vi "Teleop.vi"(10 "Match Info":T1={"Autonomous Elapsed Seconds"=0.0, "TeleOp Elapsed Seconds"=0.0, "Disabled Elapsed Seconds"=0.0, "Visited Autonomous"=FALSE, "Visited TeleOp"=FALSE, "Visited Disabled"=FALSE, "Autonomous Settings"={"Autonomous Style"=enum."Independent", "VI Refnum"=refnum}}, 11 "Call Context":T2) -> ()   [LabVIEW 2019]
doc: "This VI is called for each TeleOp packet received from the DS where the robot is not disabled. It is often used to read from the joysticks and update I/O or to update setpoints for timed control loops. It should complete and return within 20 milliseconds or it may miss DS packets."
uses:
  <vilib>/Rock Robotics/WPI/DriverStation/WPI_DriverStationDerivedRobotMode.ctl
  <vilib>/Rock Robotics/WPI/DriverStation/WPI_DriverStationMatch Info.ctl
  <vilib>/Rock Robotics/WPI/ThirdParty/Phoenix-LabVIEW/Motor Controller/Controls/CTRE_Phoenix_MotorControl_ControlMode.ctl
  <vilib>/Rock Robotics/WPI/Solenoid/WPI_SolenoidValue.ctl
  <vilib>/Rock Robotics/WPI/Utilities/WPI_GetSetVariantRefNum.vi
  <vilib>/Rock Robotics/Network Tables/NT Read Boolean.vi
  <vilib>/Rock Robotics/Network Tables/NT Read Number.vi
  <vilib>/Rock Robotics/WPI/Solenoid/WPI_SolenoidSetEnum.vi
  <vilib>/Rock Robotics/WPI/RobotDrive/WPI_RobotDriveMecanumDrive_Cartesian.vi
  <vilib>/Rock Robotics/Network Tables/NT Write Numeric Array.vi
panel:
  out "Sample Slider 0":dbl(slide) scale=0.0..5.0
  out "Sample Boolean 1":bool
  out "Sample Boolean 0":bool
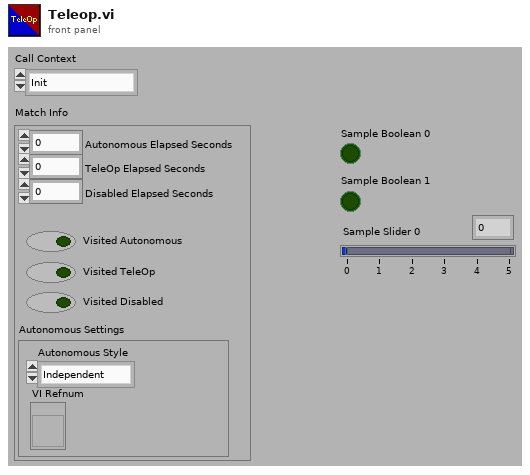
[diagram p1: front panel]
types:
  T1 = typedef "WPI_DriverStationMatch Info.ctl" = cluster{"Autonomous Elapsed Seconds":dbl, "TeleOp Elapsed Seconds":dbl, "Disabled Elapsed Seconds":dbl, "Visited Autonomous":bool, "Visited TeleOp":bool, "Visited Disabled":bool, "Autonomous Settings":cluster{"Autonomous Style":enum16{"Iterative", "Independent"}, "VI Refnum":refnum<vi>}}
  T2 = typedef "WPI_DriverStationDerivedRobotMode.ctl" = enum16{"Init", "Execute", "Stop"}
  T3 = typedef "CTRE_Phoenix_MotorControl_ControlMode.ctl" = u16
  T4 = typedef "WPI_JoystickDevRef.ctl" = cluster{"Device":T5}
  T5 = typedef "WPI_JoystickDeviceEnum.ctl" = enum16{"USB 0", "USB 1", "USB 2", "USB 3", "USB 4", "USB 5"}
  T6 = typedef "WPI_DigitalInputDevRef.ctl" = cluster{"DevStatus":errorcluster, "DIO Channel":T7}
  T7 = typedef "FPGA_DIOChannel.ctl" = enum8{"DIO 0", "DIO 1", "DIO 2", "DIO 3", "DIO 4", "DIO 5", "DIO 6", "DIO 7", "DIO 8", "DIO 9", "DIO MXP 0", "DIO MXP 1", "DIO MXP 2", "DIO MXP 3", "DIO MXP 4", "DIO MXP 5", "DIO MXP 6", "DIO MXP 7", "DIO MXP 8", "DIO MXP 9", "DIO MXP 10", "DIO MXP 11", "DIO MXP 12", "DIO MXP 13", "DIO MXP 14", "DIO MXP 15", "SPI Port CS1", "SPI Port CS2", "SPI Port CS3", "SPI Port MISO", "SPI Port MOSI", "Invalid"}
  T8 = typedef "WPI_MotorControlDeviceRef.ctl" = cluster{"DeviceStatus":errorcluster, "Type":T9, "PWM":cluster{"PWM Channel":T10, "DeadBand":T11}, "CAN":cluster{"Device Number":u8, "SetOutput VI Ref":variant, "GetOutput VI Ref":variant, "Enable VI Ref":variant, "Disable VI Ref":variant, "Data":variant}, "Invert":bool, "DIO PWM":cluster{"PWM \"Enable\" Channel":T10, "DIOChannel":T7, "PWM Rate":dbl}}
  T9 = typedef "WPI_MotorControlType.ctl" = enum16{"PWM", "CAN", "DIO PWM"}
  T10 = typedef "FPGA_DIOPWMChannel.ctl" = enum8{"PWM 0", "PWM 1", "PWM 2", "PWM 3", "PWM 4", "PWM 5", "PWM 6", "PWM 7", "PWM 8", "PWM 9", "PWM MXP 0", "PWM MXP 1", "PWM MXP 2", "PWM MXP 3", "PWM MXP 4", "PWM MXP 5", "PWM MXP 6", "PWM MXP 7", "PWM MXP 8", "PWM MXP 9", "Invalid"}
  T11 = typedef "WPI_PWMDeadband.ctl" = cluster{"Name":string, "maxPositivePwm":i32, "minPositivePwm":i32, "centerPwm":i32, "maxNegativePwm":i32, "minNegativePwm":i32, "angularRange":u16}
  T12 = typedef "WPI_RobotDriveDevRef.ctl" = cluster{"DevStatus":errorcluster, "Motors[]":T8[], "Square Inputs":bool, "Max Output":dbl}
  T13 = typedef "WPI_SolenoidDevRef.ctl" = cluster{"DevStatus":errorcluster, "Pneumatics Control Module":u8, "Forward Solenoid Channel":T14, "Reverse Solenoid Channel":T14}
  T14 = typedef "WPI_SolenoidChannel.ctl" = enum8{"Solenoid 0", "Solenoid 1", "Solenoid 2", "Solenoid 3", "Solenoid 4", "Solenoid 5", "Solenoid 6", "Solenoid 7", "Invalid"}
  T15 = typedef "WPI_SolenoidValue.ctl" = enum16{"Off", "On", "Forward", "Reverse"}
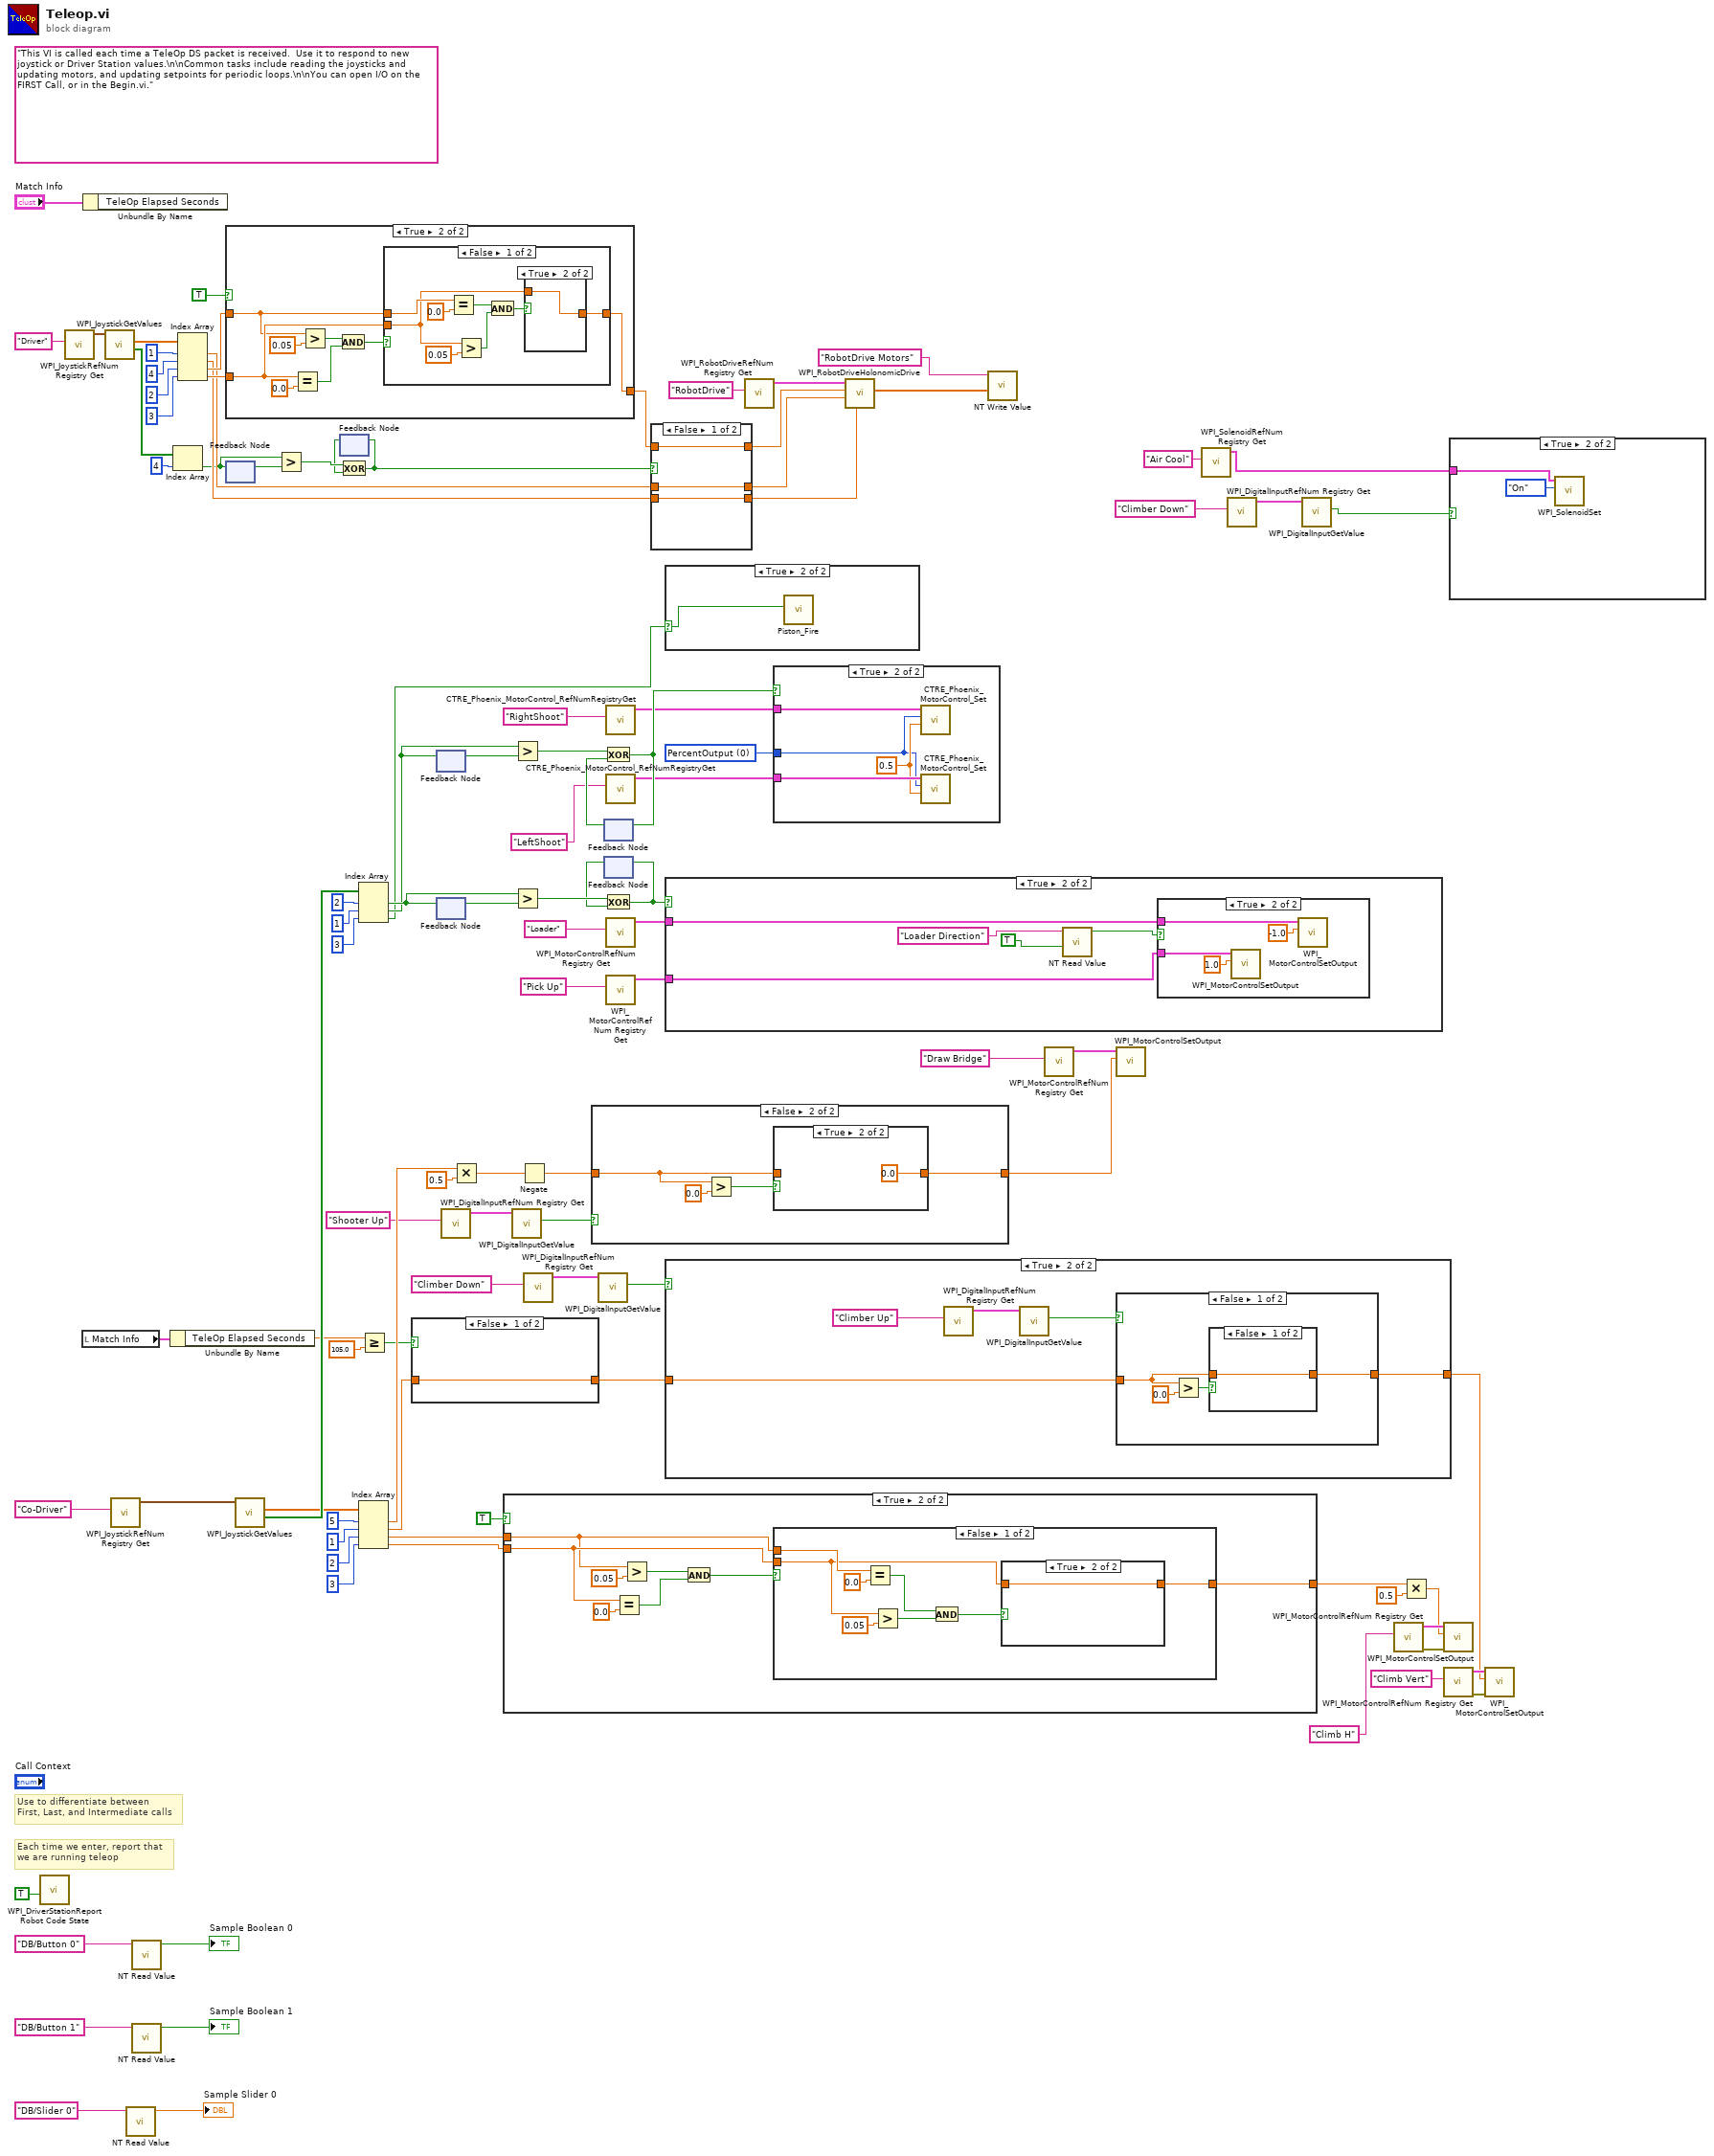
[diagram p0: block diagram]
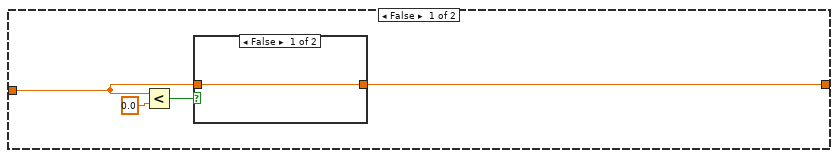
[diagram p3: hidden frame]
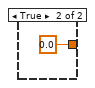
[diagram p4: hidden frame]
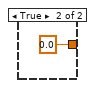
[diagram p5: hidden frame]
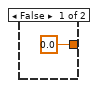
[diagram p10: hidden frame]
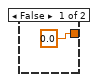
[diagram p11: hidden frame]
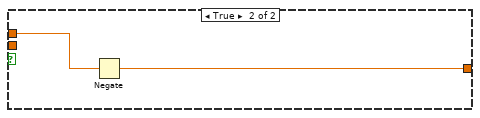
[diagram p12: hidden frame]
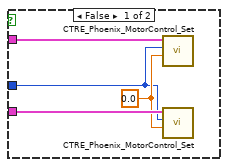
[diagram p14: hidden frame]
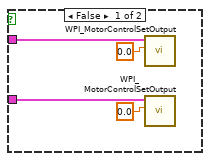
[diagram p15: hidden frame]
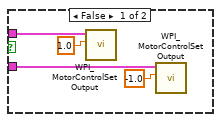
[diagram p16: hidden frame]
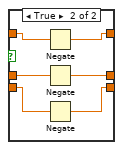
[diagram p17: hidden frame]
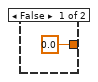
[diagram p18: hidden frame]
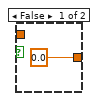
[diagram p19: hidden frame]
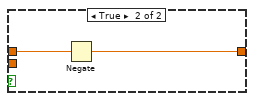
[diagram p20: hidden frame]
diagram:
  w47 = T3 0 items=["PercentOutput"=0, "Position"=1, "Velocity"=2, "Current"=3, "Follower"=5, "MotionProfile"=6, "MotionMagic"=7, "MotionProfileArc"=10, "Disabled"=15] ("Control Mode")
  (unwired) "This VI is called each time a TeleOp DS packet is received.  Use it to respond to new joystick or Driver Station values.\n\nCommon tasks include reading the joysticks and updating motors, and updating setpoints for periodic loops.\n\nYou can open I/O on the FIRST Call, or in the Begin.vi."
  # "Each time we enter, report that\nwe are running teleop"
  # "Use to differentiate between\nFirst, Last, and Intermediate calls"
  n1 = call <vilib>:"WPI_DriverStationReport Robot Code State.vi"("TeleOp"=TRUE ("Autonomous")) -> ()  [unwired: 10 in, 1 out]
  n2 = call <vilib>:"WPI_JoystickRefNum Registry Get.vi"("refnum name"="Driver") -> ("JoystickDevRef"=w99:T4)  [unwired: 1 in, 9 out]
  n3 = local read "Match Info"() -> (w27:T1)
  n4 = Unbundle By Name("Match Info") -> ()  [unwired: 1 out]
  n5 = call <vilib>:"WPI_JoystickGetValues.vi"("JoystickDevRef"=w99) -> ("Buttons"=w75:bool[], "Axes"=w97:dbl[])  [unwired: 6 in, 3 out]
  n6 = call <vilib>:"WPI_JoystickRefNum Registry Get.vi"("refnum name"="Co-Driver") -> ("JoystickDevRef"=w67:T4)  [unwired: 9 in, 1 out]
  n7 = call-poly <vilib>:"NT Read Value.vi"("Name"="DB/Slider 0" ("refnum name")) -> ("Numeric"=→"Sample Slider 0":dbl)  [unwired: 9 in, 1 out]
  n8 = call-poly <vilib>:"NT Read Value.vi"("Name"="DB/Button 0" ("refnum name")) -> ("Boolean"=→"Sample Boolean 0":bool)  [unwired: 9 in, 1 out]
  n9 = call-poly <vilib>:"NT Read Value.vi"("Name"="DB/Button 1" ("refnum name")) -> ("Boolean"=→"Sample Boolean 1":bool)  [unwired: 9 in, 1 out]
  n10 = Unbundle By Name(w27) -> ("TeleOp Elapsed Seconds"=w26:dbl)
  n11 = Index Array(array=w75, index=4) -> (element=w73:bool)
  n12 = Index Array(array=w97, index #1=1 ("index"), index #2=4 ("index"), index #3=2 ("index"), index #4=3 ("index")) -> (element #1=w80:dbl, element #2=w79:dbl, element #3=w83:dbl, element #4=w82:dbl)
  n13 = case shown="True" TRUE {
    tunnel: w83 -> [_ w106]
    tunnel: w82 -> [_ w107]
    tunnel: [0.0 w105] -> w81
    frame False {
    }
    frame True {
      n14 = Equal?(x=w107, y=0.0) -> (x = y?=w109:bool)
      n15 = Greater?(x=w106, y=0.05) -> (0:w110:bool)
      n16 = And(x=w110, y=w109) -> (x .and. y?=w108:bool)
      n17 = case shown="False" w108 {
        tunnel: w107 -> [w114 _]
        tunnel: w106 -> [w120 w124]
        tunnel: [w113 w123] -> w105
        frame False {
          n18 = Equal?(x=w120, y=0.0) -> (x = y?=w117:bool)
          n19 = Greater?(x=w114, y=0.05) -> (0:w116:bool)
          n20 = And(x=w117, y=w116) -> (x .and. y?=w115:bool)
          n21 = case shown="True" w115 {
            tunnel: w114 -> [_ w122]
            tunnel: [0.0 w122] -> w113
            frame False {
            }
            frame True {
            }
          }
        }
        frame True {
          n22 = Negate(x=w124) -> (-x=w123:dbl)
        }
      }
    }
  }
  n23 = feedback-in #1(w73) -> ()
  n24 = feedback #1() -> (w72:bool)  [unwired: 1 in]
  n25 = call <vilib>:"WPI_JoystickGetValues.vi"("JoystickDevRef"=w67) -> ("Buttons"=w66:bool[], "Axes"=w36:dbl[])  [unwired: 6 in, 3 out]
  n26 = Greater?(x=w73, y=w72) -> (0:w71:bool)
  n27 = feedback #2() -> (w70:bool)  [unwired: 1 in]
  n28 = Exclusive Or(1:w70, 2:w71) -> (0:w69:bool)
  n29 = feedback-in #2(w69) -> ()
  n30 = Index Array(array=w66, index #1=2 ("index"), index #2=1 ("index"), index #3=3 ("index")) -> (element #1=w57:bool, element #2=w52:bool, element #3=w6:bool)
  n31 = Index Array(array=w36, index #1=5 ("index"), index #2=1 ("index"), index #3=2 ("index"), index #4=3 ("index")) -> (element #1=w44:dbl, element #2=w23:dbl, element #3=w31:dbl, element #4=w32:dbl)
  n32 = Greater Or Equal?(x=w26, y=105.0) -> (x >= y?=w24:bool)
  n33 = case shown="False" w24 {
    tunnel: [w125 w126] -> w7
    tunnel: w23 -> [w125 w126]
    frame False {
    }
    frame True {
    }
  }
  n34 = feedback #3() -> (w54:bool)  [unwired: 1 in]
  n35 = feedback-in #3(w52) -> ()
  n36 = feedback-in #4(w57) -> ()
  n37 = feedback #4() -> (w64:bool)  [unwired: 1 in]
  n38 = call <vilib>:"WPI_DigitalInputRefNum Registry Get.vi"("refnum name"="Shooter Up") -> ("DigitalInputDevRef"=w17:T6)  [unwired: 9 in, 1 out]
  n39 = Multiply(x=w44, y=0.5) -> (x*y=w39:dbl)
  n40 = case shown="True" TRUE {
    tunnel: w31 -> [_ w129]
    tunnel: w32 -> [_ w130]
    tunnel: [0.0 w128] -> w20
    frame False {
    }
    frame True {
      n41 = Equal?(x=w130, y=0.0) -> (x = y?=w132:bool)
      n42 = Greater?(x=w129, y=0.05) -> (0:w133:bool)
      n43 = And(x=w133, y=w132) -> (x .and. y?=w131:bool)
      n44 = case shown="False" w131 {
        tunnel: w130 -> [w138 _]
        tunnel: w129 -> [w143 w147]
        tunnel: [w137 w146] -> w128
        frame False {
          n45 = Equal?(x=w143, y=0.0) -> (x = y?=w140:bool)
          n46 = Greater?(x=w138, y=0.05) -> (0:w139:bool)
          n47 = And(x=w140, y=w139) -> (x .and. y?=w136:bool)
          n48 = case shown="True" w136 {
            tunnel: w138 -> [_ w145]
            tunnel: [0.0 w145] -> w137
            frame False {
            }
            frame True {
            }
          }
        }
        frame True {
          n49 = Negate(x=w147) -> (-x=w146:dbl)
        }
      }
    }
  }
  n50 = call <vilib>:"WPI_DigitalInputGetValue.vi"("DigitalInputDevRef"=w17) -> ("Value"=w16:bool)  [unwired: 8 in, 2 out]
  n51 = Greater?(x=w52, y=w54) -> (0:w55:bool)
  n52 = Greater?(x=w57, y=w64) -> (0:w63:bool)
  n53 = Negate(x=w39) -> (-x=w15:dbl)
  n54 = call <vilib>:"WPI_DigitalInputRefNum Registry Get.vi"("refnum name"="Climber Down") -> ("DigitalInputDevRef"=w10:T6)  [unwired: 9 in, 1 out]
  n55 = case shown="False" w16 {
    tunnel: w15 -> [w148 w149]
    tunnel: [w148 w150] -> w14
    frame True {
    }
    frame False {
      n56 = Greater?(x=w149, y=0.0) -> (0:w152:bool)
      n57 = case shown="True" w152 {
        tunnel: [w153 0.0] -> w150
        tunnel: w149 -> [w153 _]
        frame False {
        }
        frame True {
        }
      }
    }
  }
  n58 = call <vilib>:"WPI_DigitalInputGetValue.vi"("DigitalInputDevRef"=w10) -> ("Value"=w9:bool)  [unwired: 8 in, 2 out]
  n59 = feedback #5() -> (w56:bool)  [unwired: 1 in]
  n60 = Exclusive Or(1:w56, 2:w55) -> (0:w53:bool)
  n61 = feedback-in #5(w53) -> ()
  n62 = feedback #6() -> (w62:bool)  [unwired: 1 in]
  n63 = Exclusive Or(1:w62, 2:w63) -> (0:w61:bool)
  n64 = feedback-in #6(w61) -> ()
  n65 = call <vilib>:"CTRE_Phoenix_MotorControl_RefNumRegistryGet.vi"("refnum name"="RightShoot") -> ("PhoenixMotorControlDevRef"=w48:T8)  [unwired: 9 in, 1 out]
  n66 = call <vilib>:"CTRE_Phoenix_MotorControl_RefNumRegistryGet.vi"("refnum name"="LeftShoot") -> ("PhoenixMotorControlDevRef"=w49:T8)  [unwired: 9 in, 1 out]
  n67 = call <vilib>:"WPI_MotorControlRefNum Registry Get.vi"("refnum name"="Loader") -> ("MotorControlDevRef"=w60:T8)  [unwired: 9 in, 1 out]
  n68 = call <vilib>:"WPI_MotorControlRefNum Registry Get.vi"("refnum name"="Pick Up") -> ("MotorControlDevRef"=w41:T8)  [unwired: 9 in, 1 out]
  n69 = case shown="False" w69 {
    tunnel: w81 -> [w157 w159]
    tunnel: w80 -> [w156 w161]
    tunnel: w79 -> [w155 w163]
    tunnel: [w157 w158] -> w78
    tunnel: [w156 w160] -> w77
    tunnel: [w155 w162] -> w76
    frame False {
    }
    frame True {
      n70 = Negate(x=w159) -> (-x=w158:dbl)
      n71 = Negate(x=w161) -> (-x=w160:dbl)
      n72 = Negate(x=w163) -> (-x=w162:dbl)
    }
  }
  n73 = case shown="True" w6 {
    selector: w6 -> [_ w164]
    frame False {
    }
    frame True {
      n74 = call "Piston_Fire.vi"("Fire?"=w164) -> ()  [unwired: 11 in]
    }
  }
  n75 = case shown="True" w61 {
    tunnel: w60 -> [w168 w173]
    tunnel: w41 -> [w165 w169]
    frame False {
      n76 = call <vilib>:"WPI_MotorControlSetOutput.vi"("Output"=0.0, "MotorControlDevRef"=w168) -> ()  [unwired: 7 in, 3 out]
      n77 = call <vilib>:"WPI_MotorControlSetOutput.vi"("Output"=0.0, "MotorControlDevRef"=w165) -> ()  [unwired: 7 in, 3 out]
    }
    frame True {
      n78 = call-poly <vilib>:"NT Read Value.vi"("Default Value"=TRUE, "Name"="Loader Direction") -> ("Boolean"=w170:bool)  [unwired: 8 in, 1 out]
      n79 = case shown="True" w170 {
        tunnel: w173 -> [w176 w181]
        tunnel: w169 -> [w174 w178]
        frame False {
          n80 = call <vilib>:"WPI_MotorControlSetOutput.vi"("Output"=1.0, "MotorControlDevRef"=w176) -> ()  [unwired: 7 in, 3 out]
          n81 = call <vilib>:"WPI_MotorControlSetOutput.vi"("Output"=-1.0, "MotorControlDevRef"=w174) -> ()  [unwired: 7 in, 3 out]
        }
        frame True {
          n82 = call <vilib>:"WPI_MotorControlSetOutput.vi"("Output"=1.0, "MotorControlDevRef"=w178) -> ()  [unwired: 7 in, 3 out]
          n83 = call <vilib>:"WPI_MotorControlSetOutput.vi"("Output"=-1.0, "MotorControlDevRef"=w181) -> ()  [unwired: 7 in, 3 out]
        }
      }
    }
  }
  n84 = case shown="True" w9 {
    tunnel: [w182 w189] -> w8
    tunnel: w7 -> [w183 w188]
    frame False {
      n85 = Less?(x=w183, y=0.0) -> (x < y?=w185:bool)
      n86 = case shown="False" w185 {
        tunnel: w183 -> [w186 _]
        tunnel: [w186 0.0] -> w182
        frame False {
        }
        frame True {
        }
      }
    }
    frame True {
      n87 = call <vilib>:"WPI_DigitalInputRefNum Registry Get.vi"("refnum name"="Climber Up") -> ("DigitalInputDevRef"=w191:T6)  [unwired: 9 in, 1 out]
      n88 = call <vilib>:"WPI_DigitalInputGetValue.vi"("DigitalInputDevRef"=w191) -> ("Value"=w190:bool)  [unwired: 8 in, 2 out]
      n89 = case shown="False" w190 {
        tunnel: [w194 w199] -> w189
        tunnel: w188 -> [w193 w199]
        frame False {
          n90 = Greater?(x=w193, y=0.0) -> (0:w195:bool)
          n91 = case shown="False" w195 {
            tunnel: [w197 0.0] -> w194
            tunnel: w193 -> [w197 _]
            frame False {
            }
            frame True {
            }
          }
        }
        frame True {
        }
      }
    }
  }
  n92 = call <vilib>:"WPI_RobotDriveRefNum Registry Get.vi"("refnum name"="RobotDrive") -> ("RobotDriveDevRef"=w101:T12)  [unwired: 1 in, 9 out]
  n93 = case shown="True" w53 {
    tunnel: w49 -> [w203 w207]
    tunnel: w48 -> [w202 w206]
    tunnel: w47 -> [w200 w204]
    frame False {
      w201 = 0.0 ("Output")
      n94 = call <vilib>:"CTRE_Phoenix_MotorControl_Set.vi"("Output"=w201, "Control Mode"=w200, "PhoenixMotorControlDevRef"=w202) -> ()  [unwired: 7 in, 2 out]
      n95 = call <vilib>:"CTRE_Phoenix_MotorControl_Set.vi"("Output"=w201, "Control Mode"=w200, "PhoenixMotorControlDevRef"=w203) -> ()  [unwired: 7 in, 2 out]
    }
    frame True {
      w205 = 0.5 ("Output")
      n96 = call <vilib>:"CTRE_Phoenix_MotorControl_Set.vi"("Output"=w205, "Control Mode"=w204, "PhoenixMotorControlDevRef"=w206) -> ()  [unwired: 7 in, 2 out]
      n97 = call <vilib>:"CTRE_Phoenix_MotorControl_Set.vi"("Output"=w205, "Control Mode"=w204, "PhoenixMotorControlDevRef"=w207) -> ()  [unwired: 7 in, 2 out]
    }
  }
  n98 = call-poly <vilib>:"WPI_RobotDriveHolonomicDrive.vi"("Rotation"=w76, "Y"=w77, "X"=w78, "RobotDriveDevRef"=w101) -> ("Motor Values"=w90:dbl[])  [unwired: 5 in, 2 out]
  n99 = call-poly <vilib>:"NT Write Value.vi"("Numeric Array"=w90, "Name"="RobotDrive Motors") -> ()  [unwired: 9 in, 1 out]
  n100 = call <vilib>:"WPI_MotorControlRefNum Registry Get.vi"("refnum name"="Draw Bridge") -> ("MotorControlDevRef"=w13:T8)  [unwired: 9 in, 1 out]
  n101 = call <vilib>:"WPI_MotorControlSetOutput.vi"("Output"=w14, "MotorControlDevRef"=w13) -> ()  [unwired: 7 in, 3 out]
  n102 = call <vilib>:"WPI_SolenoidRefNum Registry Get.vi"("refnum name"="Air Cool") -> ("SolenoidDevRef"=w3:T13)  [unwired: 9 in, 1 out]
  n103 = call <vilib>:"WPI_DigitalInputRefNum Registry Get.vi"("refnum name"="Climber Down") -> ("DigitalInputDevRef"=w4:T6)  [unwired: 9 in, 1 out]
  n104 = call <vilib>:"WPI_DigitalInputGetValue.vi"("DigitalInputDevRef"=w4) -> ("Value"=w1:bool)  [unwired: 8 in, 2 out]
  n105 = call <vilib>:"WPI_MotorControlRefNum Registry Get.vi"("refnum name"="Climb H") -> ("error out"=w22:errorcluster, "MotorControlDevRef"=w29:T8)  [unwired: 9 in]
  n106 = Multiply(x=w20, y=0.5) -> (x*y=w18:dbl)
  n107 = call <vilib>:"WPI_MotorControlSetOutput.vi"("error in (no error)"=w22, "Output"=w18, "MotorControlDevRef"=w29) -> ()  [unwired: 6 in, 3 out]
  n108 = call <vilib>:"WPI_MotorControlRefNum Registry Get.vi"("refnum name"="Climb Vert") -> ("error out"=w21:errorcluster, "MotorControlDevRef"=w38:T8)  [unwired: 9 in]
  n109 = case shown="True" w1 {
    tunnel: w3 -> [_ w209]
    frame False {
    }
    frame True {
      n110 = call-poly <vilib>:"WPI_SolenoidSet.vi"("Value"=WPI_SolenoidValue."On", "SolenoidDevRef"=w209) -> ()  [unwired: 8 in, 2 out]
    }
  }
  n111 = call <vilib>:"WPI_MotorControlSetOutput.vi"("error in (no error)"=w21, "Output"=w8, "MotorControlDevRef"=w38) -> ()  [unwired: 6 in, 3 out]
